vi "Fit VI window to Panel Center.vi"(4 "Error In":errorcluster, 6 "Panel Ref":refnum<vi>, 7 "VI Ref":refnum<vi>) -> (0 "Error Out":errorcluster, 3 "dup VI Ref":refnum<vi>)   [LabVIEW 2017, in "csm-ui-support.lvlib"]
doc: "This VI is designed to center a callee VI's window in a caller VI's window.\n\nAuthored by Brandon Steele\nsupport@mooregoodideas.com\nwww.mooregoodideas.com\n\nCopyright (c) 2010, Moore Good Ideas, Inc.\n\nAll rights reserved.\n\nRedistribution and use in source and binary forms, with or without modification, are permitted provided that the following conditions are met:\n\n * Redistributions of source code must retain the above copyright notice, this list of conditions and the following disclaimer.\n * Redistributions in binary form must reproduce the above copyright notice, this list of conditions and the following disclaimer in the documentation and/or other materials provided with the distribution.\n * Neither the name of Moore Good Ideas, Inc. nor the names of its contributors may be used to endorse or promote products derived from this software without specific prior written permission.\n\nTHIS SOFTWARE IS PROVIDED BY THE COPYRIGHT HOLDERS AND CONTRIBUTORS \"AS IS\" AND ANY EXPRESS OR IMPLIED WARRANTIES, INCLUDING, BUT NOT LIMITED TO, THE IMPLIED WARRANTIES OF MERCHANTABILITY AND FITNESS FOR A PARTICULAR PURPOSE ARE DISCLAIMED. IN NO EVENT SHALL THE COPYRIGHT OWNER OR CONTRIBUTORS BE LIABLE FOR ANY DIRECT, INDIRECT, INCIDENTAL, SPECIAL, EXEMPLARY, OR CONSEQUENTIAL DAMAGES (INCLUDING, BUT NOT LIMITED TO, PROCUREMENT OF SUBSTITUTE GOODS OR SERVICES; LOSS OF USE, DATA, OR PROFITS; OR BUSINESS INTERRUPTION) HOWEVER CAUSED AND ON ANY THEORY OF LIABILITY, WHETHER IN CONTRACT, STRICT LIABILITY, OR TORT (INCLUDING NEGLIGENCE OR OTHERWISE) ARISING IN ANY WAY OUT OF THE USE OF THIS SOFTWARE, EVEN IF ADVISED OF THE POSSIBILITY OF SUCH DAMAGE."
uses:
  csm-ui-support.lvlib
panel:
  in  "Pane Ref":refnum<vi>
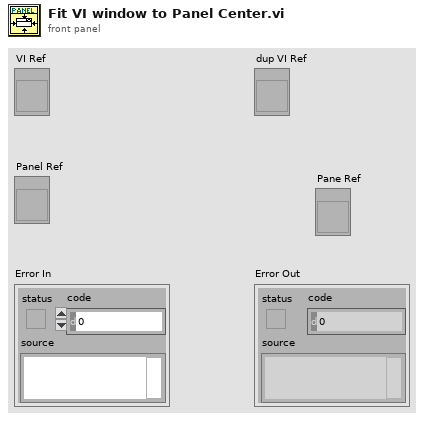
[diagram p1: front panel]
types:
  T1 = typedef "LVRectTypeDef.ctl" = cluster{"Left":i16, "Top":i16, "Right":i16, "Bottom":i16}
  T2 = cluster{"left":i16, "top":i16, "right":i16, "bottom":i16}
  T3 = typedef "LVAllMonitorsDisplayTypeDef.ctl" = cluster{"Bounds":cluster{"Left":i16, "Top":i16, "Right":i16, "Bottom":i16}, "Depth":i16}[]
  T4 = cluster{"Left":i16, "Top":i16, "Right":i16, "Bottom":i16}
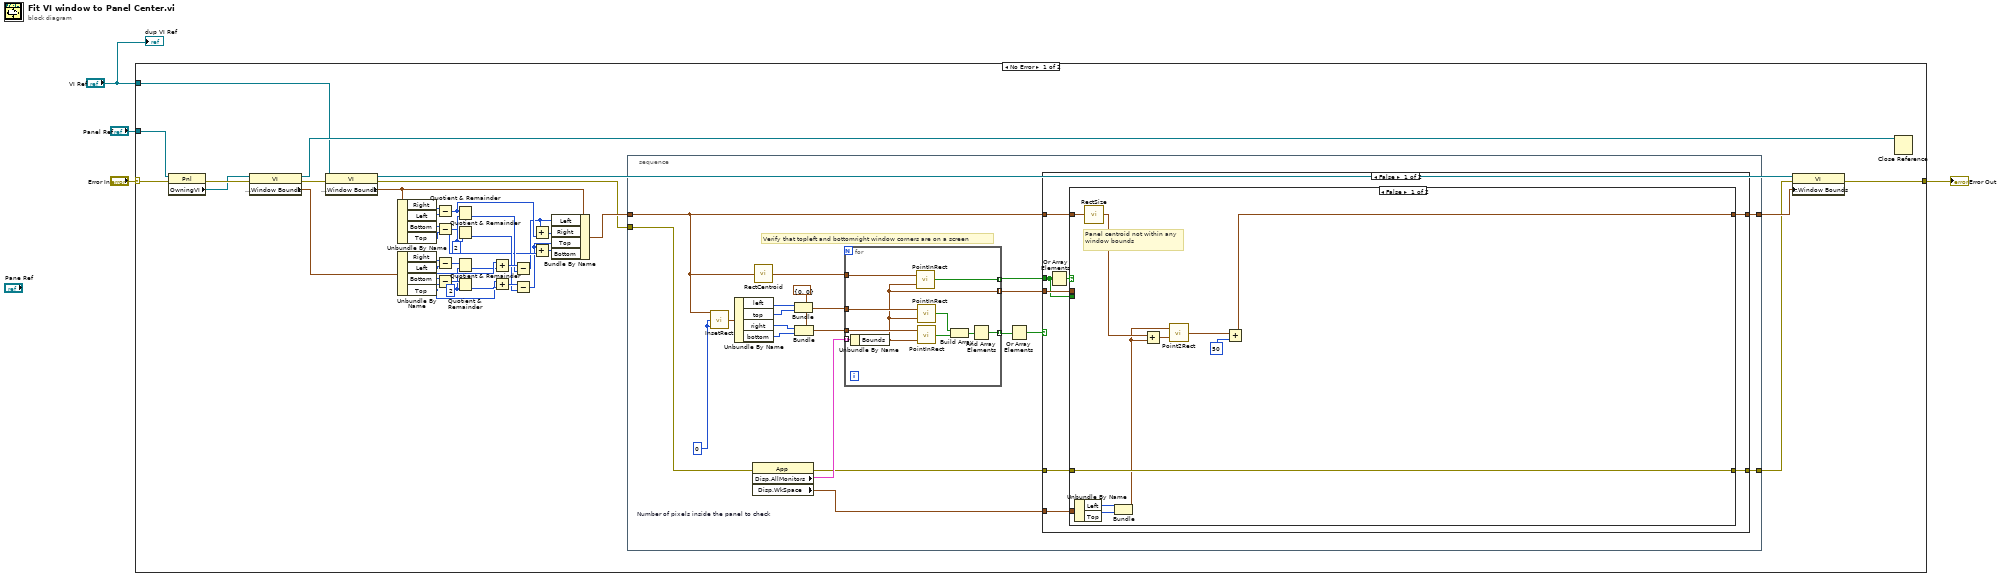
[diagram p0: block diagram]
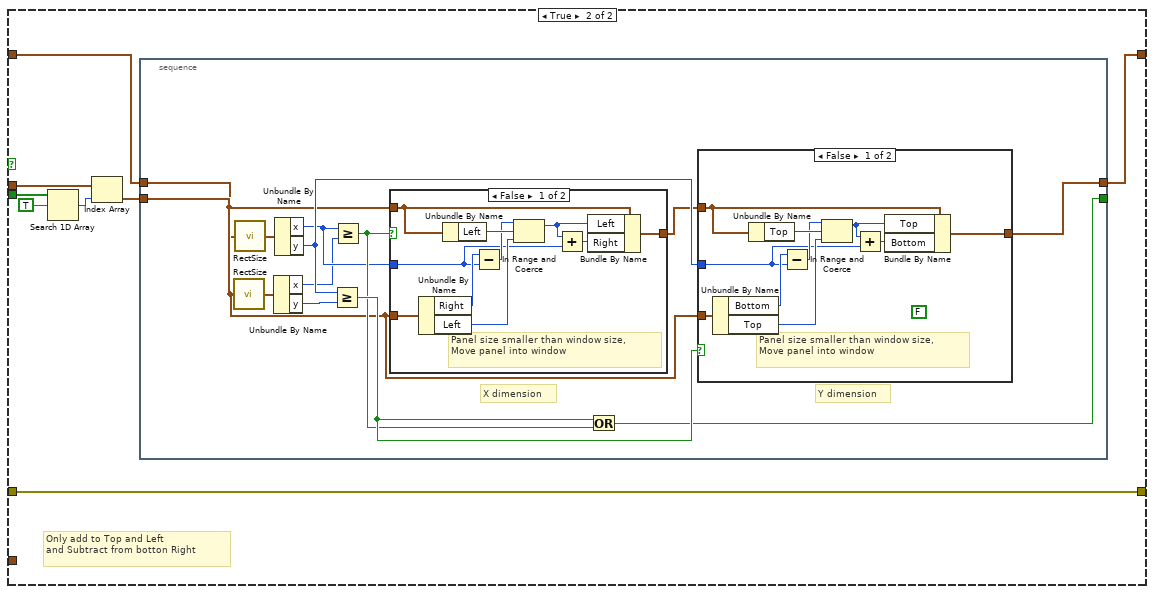
[diagram p2: hidden frame]
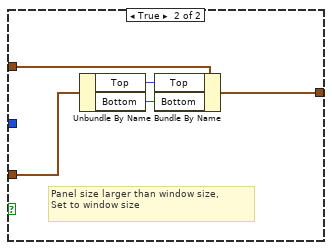
[diagram p3: hidden frame]
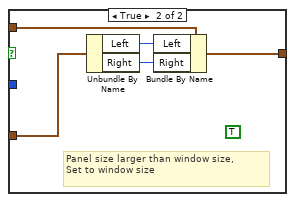
[diagram p4: hidden frame]
diagram:
  n1 = case shown="No Error" "Error In" {
    selector: "Error In" -> [w9 w147]
    tunnel: [w43 w147] -> w4
    tunnel: "Panel Ref" -> [w6 _]
    tunnel: "VI Ref" -> [w5 _]
    frame No Error {
      w36 = i16 2 ("y")
      w20 = i16 2 ("y")
      n2 = property class="Pnl"(reference=w6, error in=w9) -> (error out=w8:errorcluster, "OwningVI"=w7:refnum<vi>)  [unwired: 1 out]
      n3 = property class="VI"(reference=w7, error in=w8) -> (reference out=w19:refnum<vi>, error out=w37:errorcluster, "Front Panel Window:Window Bounds"=w42:T1)
      n4 = property class="VI"(reference=w5, error in=w37) -> (reference out=w23:refnum<vi>, error out=w11:errorcluster, "Front Panel Window:Window Bounds"=w14:T1)
      n5 = Unbundle By Name(w14) -> ("Right"=w32:i16, "Left"=w33:i16, "Bottom"=w34:i16, "Top"=w35:i16)
      n6 = Unbundle By Name(w42) -> ("Right"=w41:i16, "Left"=w31:i16, "Bottom"=w40:i16, "Top"=w28:i16)
      n7 = Subtract(x=w32, y=w33) -> (x-y=w22:i16)
      n8 = Subtract(x=w34, y=w35) -> (x-y=w21:i16)
      n9 = Subtract(x=w41, y=w31) -> (x-y=w39:i16)
      n10 = Subtract(x=w40, y=w28) -> (x-y=w38:i16)
      n11 = Quotient & Remainder(x=w22, y=w36) -> (floor(x/y)=w26:i16)  [unwired: 1 out]
      n12 = Quotient & Remainder(x=w21, y=w36) -> (floor(x/y)=w24:i16)  [unwired: 1 out]
      n13 = Quotient & Remainder(x=w39, y=w20) -> (floor(x/y)=w30:i16)  [unwired: 1 out]
      n14 = Quotient & Remainder(x=w38, y=w20) -> (floor(x/y)=w29:i16)  [unwired: 1 out]
      n15 = Add(x=w31, y=w30) -> (x+y=w27:i16)
      n16 = Add(x=w28, y=w29) -> (x+y=w25:i16)
      n17 = Subtract(x=w27, y=w26) -> (x-y=w17:i16)
      n18 = Subtract(x=w25, y=w24) -> (x-y=w16:i16)
      n19 = Add(x=w17, y=w22) -> (x+y=w15:i16)
      n20 = Add(x=w16, y=w21) -> (x+y=w18:i16)
      n21 = Bundle By Name(cluster=w14, "Left"=w17, "Right"=w15, "Top"=w16, "Bottom"=w18) -> (w13:T1)
      n22 = stacked-sequence {
        tunnel: [w54] -> w10
        tunnel: [w45] -> w12
        tunnel: w11 -> [w47]
        tunnel: w13 -> [w61]
        frame #0 {
          w56 = i16 0  # Number of pixels inside the panel to check
          w60 = cluster{"x":i16, "y":i16} {"x"=0, "y"=0} ("point")
          # "Verify that topleft and bottomright window corners are on a screen"
          n23 = call <vilib>:"InsetRect.vi"("dv"=w56, "dh"=w56, "rect"=w61) -> ("inset rect"=w50:T2)
          n24 = Unbundle By Name(w50) -> ("left"=w48:i16, "top"=w49:i16, "right"=w57:i16, "bottom"=w58:i16)
          n25 = property class="App"(error in=w47) -> (error out=w44:errorcluster, "Disp.AllMonitors"=w46:T3, "Disp.WkSpace"=w55:T1)  [unwired: 1 in, 1 out]
          n26 = call <vilib>:"RectCentroid.vi"("rect"=w61) -> ("point"=w62:cluster{"x":i16, "y":i16})
          n27 = Bundle(cluster=w60, "x"=w48, "y"=w49) -> (w51:cluster{"x":i16, "y":i16})
          n28 = Bundle(cluster=w60, "x"=w57, "y"=w58) -> (w59:cluster{"x":i16, "y":i16})
          n29 = for {
            tunnel: w46 -> [w146] mode=indexing
            tunnel: w51 -> [w145]
            tunnel: [w141] -> w52 mode=indexing
            tunnel: w59 -> [w140]
            tunnel: w62 -> [w139]
            tunnel: [w138] -> w63 mode=indexing
            tunnel: [w137] -> w64 mode=indexing
            n30 = Unbundle By Name(w146) -> ("Bounds"=w137:T4)
            n31 = call <vilib>:"PointInRect.vi"("rect"=w137, "point"=w139) -> ("pt in rect"=w138:bool)
            n32 = call <vilib>:"PointInRect.vi"("rect"=w137, "point"=w145) -> ("pt in rect"=w144:bool)
            n33 = call <vilib>:"PointInRect.vi"("rect"=w137, "point"=w140) -> ("pt in rect"=w143:bool)
            n34 = Build Array(w144, w143) -> (w142:bool[])
            n35 = And Array Elements(Boolean array=w142) -> (logical AND=w141:bool)
          }
          n36 = Or Array Elements(Boolean array=w52) -> (logical OR=w53:bool)
          n37 = case shown="False" w53 {
            tunnel: w44 -> [w67 w136]
            tunnel: [w66 w136] -> w54
            tunnel: w61 -> [w71 w135]
            tunnel: [w70 w135] -> w45
            tunnel: w55 -> [w72 _]
            tunnel: w63 -> [w65 _]
            tunnel: w64 -> [w68 _]
            frame False {
              n38 = Or Array Elements(Boolean array=w65) -> (logical OR=w69:bool)
              n39 = case shown="False" w69 {
                tunnel: w72 -> [w83 _]
                tunnel: w71 -> [w79 w86]
                tunnel: [w77 w84] -> w70
                tunnel: w68 -> [_ w88]
                tunnel: w67 -> [w76 w91]
                tunnel: [w76 w91] -> w66
                tunnel: w65 -> [_ w90]
                frame False {
                  # "Panel centroid not within any\nwindow bounds"
                  n40 = Unbundle By Name(w83) -> ("Left"=w82:i16, "Top"=w81:i16)
                  n41 = call <vilib>:"RectSize.vi"("rect"=w79) -> ("point"=w75:cluster{"x":i16, "y":i16})
                  n42 = Bundle("Left"=w82, "Top"=w81) -> (w73:cluster{"Left":i16, "Top":i16})  [unwired: 1 in]
                  n43 = Add(x=w75, y=w73) -> (x+y=w74:cluster{i16, i16})
                  n44 = call <vilib>:"Point2Rect.vi"("point b"=w74, "point a"=w73) -> ("rect"=w78:T2)
                  n45 = Add(x=w78, y=i16 50) -> (x+y=w77:T2)
                }
                frame True {
                  # "Only add to Top and Left\nand Subtract from botton Right"
                  n46 = Search 1D Array(1D array=w90, element=TRUE) -> (index of element=w87:i32)  [unwired: 1 in]
                  n47 = Index Array(array=w88, index=w87) -> (element=w85:T4)
                  n48 = stacked-sequence {
                    tunnel: [w92] -> _
                    tunnel: [w102] -> w84
                    tunnel: w85 -> [w101]
                    tunnel: w86 -> [w93]
                    frame #0 {
                      # "X dimension"
                      # "Y dimension"
                      n49 = call <vilib>:"RectSize.vi"("rect"=w101) -> ("point"=w95:cluster{"x":i16, "y":i16})
                      n50 = call <vilib>:"RectSize.vi"("rect"=w93) -> ("point"=w94:cluster{"x":i16, "y":i16})
                      n51 = Unbundle By Name(w95) -> ("x"=w96:i16, "y"=w99:i16)
                      n52 = Unbundle By Name(w94) -> ("x"=w97:i16, "y"=w100:i16)
                      n53 = Greater Or Equal?(x=w100, y=w99) -> (x >= y?=w104:bool)
                      n54 = Greater Or Equal?(x=w97, y=w96) -> (x >= y?=w103:bool)
                      n55 = case shown="False" w103 {
                        tunnel: w101 -> [w129 w130]
                        tunnel: w93 -> [w121 w131]
                        tunnel: w97 -> [w122 _]
                        tunnel: [w120 w132] -> w98
                        frame False {
                          # "Panel size smaller than window size,\nMove panel into window"
                          n56 = Unbundle By Name(w129) -> ("Right"=w125:i16, "Left"=w127:i16)
                          n57 = Unbundle By Name(w121) -> ("Left"=w128:i16)
                          n58 = Subtract(x=w125, y=w122) -> (x-y=w126:i16)
                          n59 = In Range and Coerce(upper limit=w126, x=w128, lower limit=w127) -> (coerced(x)=w124:i16)  [unwired: 1 out]
                          n60 = Add(x=w124, y=w122) -> (x+y=w123:i16)
                          n61 = Bundle By Name(cluster=w121, "Left"=w124, "Right"=w123) -> (w120:T1)
                        }
                        frame True {
                          (unwired) TRUE
                          # "Panel size larger than window size,\nSet to window size"
                          n62 = Unbundle By Name(w130) -> ("Left"=w134:i16, "Right"=w133:i16)
                          n63 = Bundle By Name(cluster=w131, "Left"=w134, "Right"=w133) -> (w132:T1)
                        }
                      }
                      n64 = Or(x=w104, y=w103) -> (x .or. y?=w92:bool)
                      n65 = case shown="False" w104 {
                        tunnel: w101 -> [w114 w119]
                        tunnel: w98 -> [w106 w115]
                        tunnel: w100 -> [w107 _]
                        tunnel: [w105 w116] -> w102
                        frame False {
                          (unwired) FALSE
                          # "Panel size smaller than window size,\nMove panel into window"
                          n66 = Unbundle By Name(w114) -> ("Bottom"=w110:i16, "Top"=w112:i16)
                          n67 = Unbundle By Name(w106) -> ("Top"=w113:i16)
                          n68 = Subtract(x=w110, y=w107) -> (x-y=w111:i16)
                          n69 = In Range and Coerce(upper limit=w111, x=w113, lower limit=w112) -> (coerced(x)=w109:i16)  [unwired: 1 out]
                          n70 = Add(x=w109, y=w107) -> (x+y=w108:i16)
                          n71 = Bundle By Name(cluster=w106, "Top"=w109, "Bottom"=w108) -> (w105:T1)
                        }
                        frame True {
                          # "Panel size larger than window size,\nSet to window size"
                          n72 = Unbundle By Name(w119) -> ("Top"=w118:i16, "Bottom"=w117:i16)
                          n73 = Bundle By Name(cluster=w115, "Top"=w118, "Bottom"=w117) -> (w116:T1)
                        }
                      }
                    }
                  }
                }
              }
            }
            frame True {
            }
          }
        }
      }
      n74 = property class="VI"(reference=w23, error in=w10, "Front Panel Window:Window Bounds"=w12) -> (error out=w43:errorcluster)  [unwired: 1 out]
      n75 = Close Reference(reference=w19) -> ()  [unwired: 1 in, 1 out]
    }
    frame Error {
    }
  }
  "Error Out" <- w4
  "dup VI Ref" <- "VI Ref"
